vi "AprilTag Target Package Code 1.vi"() -> ()   [LabVIEW 2023]
uses:
  Camera Info.ctl
  State Machine/AprialTag Main Cluster.ctl
  State Machine/AprialTag States.ctl
  <vilib>/vision/Image Controls.llb/IMAQ Image.ctl
  Steam Type.ctl
  Camera Set Up/Event Setup Types.ctl
  <vilib>/Utility/config.llb/Read Key (String).vi
  <vilib>/Utility/config.llb/Write Key (String).vi
  <vilib>/Utility/config.llb/NI_LVConfig.lvlib
panel:
  in  "Main":enum32{"Page 1", "Page 2"}(tab)
  out "Target Pitch":dbl[](array[numeric]) caption="Tag Pitch (deg)" format="%.1f"
  out "Target Yaw":dbl[](array[numeric]) caption="Tag Yaw (deg)" format="%.1f"
  out "Tag ID":dbl[](array[numeric]) caption="Tag Number"
  out "Image":T1(plugin-control)
  in  "Camera Name":string="cam0"
  in  "Settings":bool
  in  "Save":bool
  in  "Tools":bool
  out "AprilTag Fps":dbl format="%#.0f"
  out "Distance":dbl[](array[numeric]) caption="Tag Distance (in)" format="%.1f"
  out "Angle":dbl[](array[numeric]) caption="Center Angle (deg)" format="%.1f"
  in  "Home":bool
  in  "Robot Calibration Cluster":T2={"Camera Height on robot (in)"=9.5, "Camera Angle on the robot (deg)"=2.5, "Camera FOV Top to Bottom View Angle (deg)"=26.5, "Camera FOV Left to Right View Angle (deg)"=68.5, "Target size (in)"=6.5, "Distance to front of bumper (in)"=9.75, "Focal Length (mm)"=10.0} {"Camera FOV Left to Right View Angle (deg)" format="%#_13g"; "Focal Length (mm)" format="%#_13g"; "Distance to front of bumper (in)" format="%#_13g"; "Target size (in)" format="%#_13g"; "Camera FOV Top to Bottom View Angle (deg)" format="%#_13g"; "Camera Angle on the robot (deg)" format="%#_13g"; "Camera Height on robot (in)" format="%#_13g"}
  # "Edit the camera name to the camera that you are going to use for this target package"
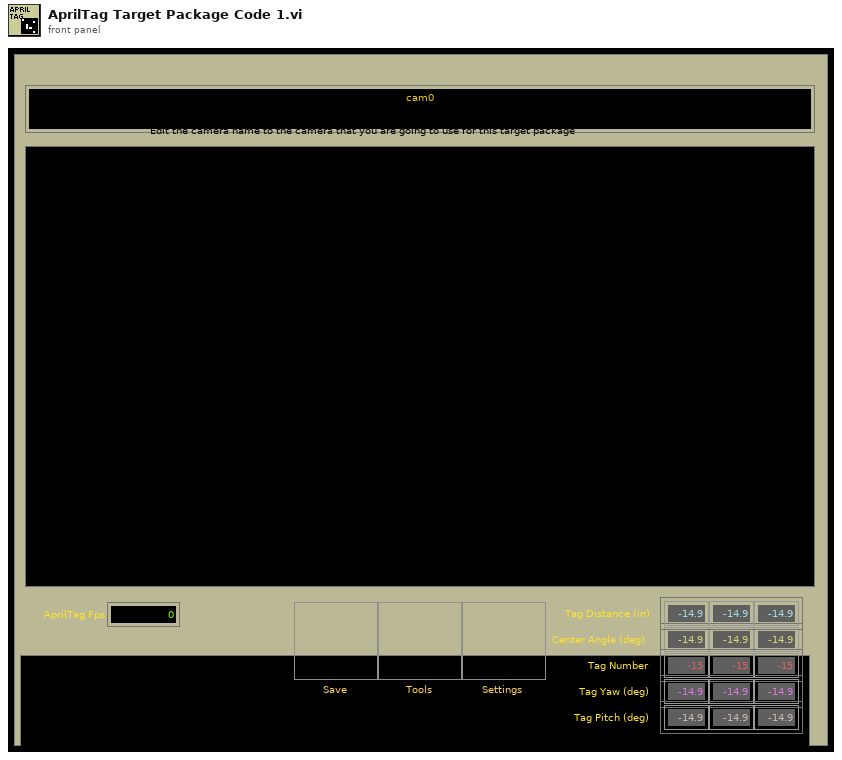
[diagram p1: front panel]
types:
  T1 = typedef "IMAQ Image.ctl" = refnum<image>
  T2 = typedef "Camera Info.ctl" = cluster{"Camera Height on robot (in)":dbl, "Camera Angle on the robot (deg)":dbl, "Camera FOV Top to Bottom View Angle (deg)":dbl, "Camera FOV Left to Right View Angle (deg)":dbl, "Target size (in)":dbl, "Distance to front of bumper (in)":dbl, "Focal Length (mm)":dbl}
  T3 = typedef "AprialTag States.ctl" = enum16{"Message Dispatcher", "INI", "Open", "Save", "Exit"}
  T4 = typedef "AprialTag Main Cluster.ctl" = cluster{"AprilTage FIFO":T3[], "Camera Name":string, "AprilTag path":path, "Control Ref's":refnum<vi>[], "Calibration Mask":T1, "Main Image":T1, "Timeout":i32, "EDIT Settings":bool, "Calibration path":path, "Camera Number":dbl}
  T5 = typedef "Steam Type.ctl" = enum8{"Unknown", "Apriltag", "Algae", "Coral"}
  T6 = typedef "Event Setup Types.ctl" = enum16{"Default", "Camera Loop Started", "Close Settings", "GreyScale", "Open Front Panel", "Save Data", "Exit"}
  T7 = cluster{"tag ID":i32, "Center":cluster{"X":dbl, "Y":dbl}, "homography matrix":dbl[], "decision margin":dbl, "Hamming Dist":i32, "corner points":cluster{"X":dbl, "Y":dbl}[], "Tag Family":string}[]
  T8 = typedef "AprilTag Target Fields.ctl" = cluster{"diameter points":cluster{"first point":cluster{"x":dbl, "y":dbl}, "projected point":cluster{"x":dbl, "y":dbl}}, "normalized center":cluster{"x":dbl, "y":dbl}, "Overall Score":dbl, "Distance (ft)":dbl, "Offset Angle":dbl, "Tag corner points":cluster{"X":dbl, "Y":dbl}[], "Tag Center":cluster{"X":dbl, "Y":dbl}, "Tag Yaw":dbl, "Tag Pitch":dbl, "Target Roll (deg)":dbl, "AprilTag Number":i32}
  T9 = typedef "Image Type" = u32
  T10 = typedef "NI_LVConfig.lvlib/Config Data RefNum.ctl" = refnum<k1>
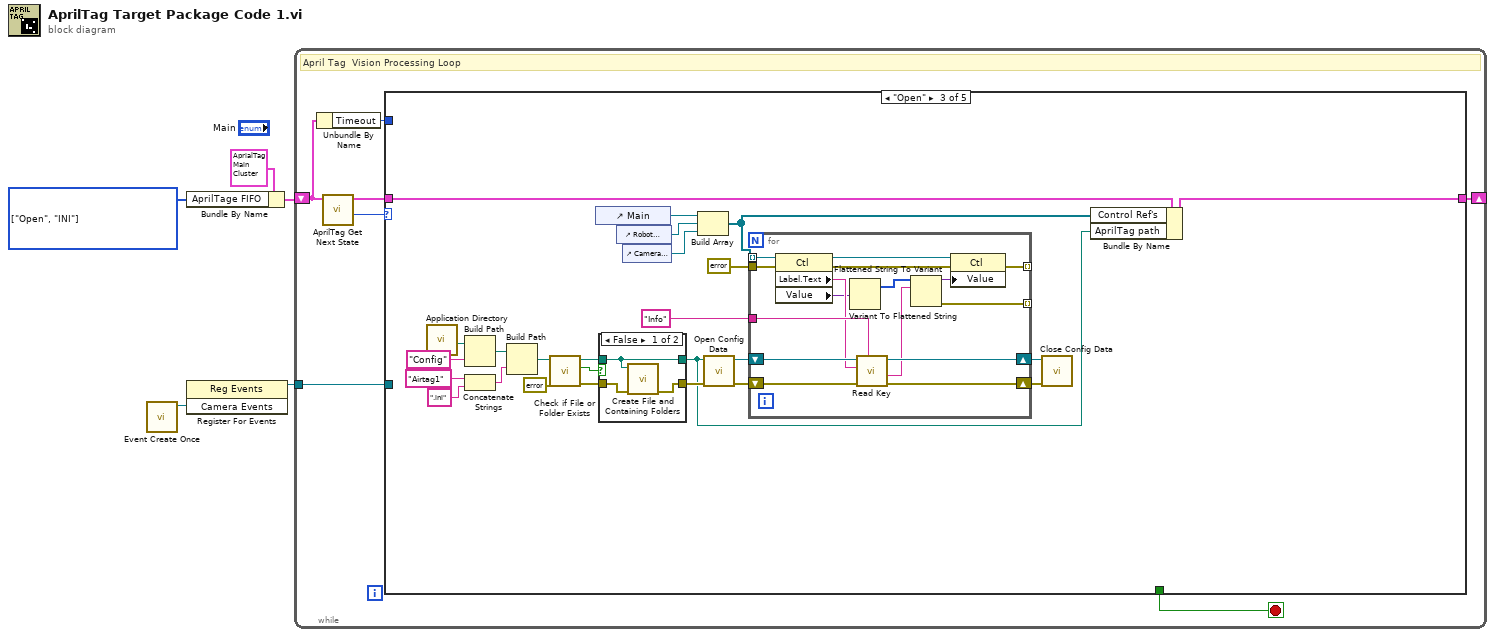
[diagram p0: block diagram]
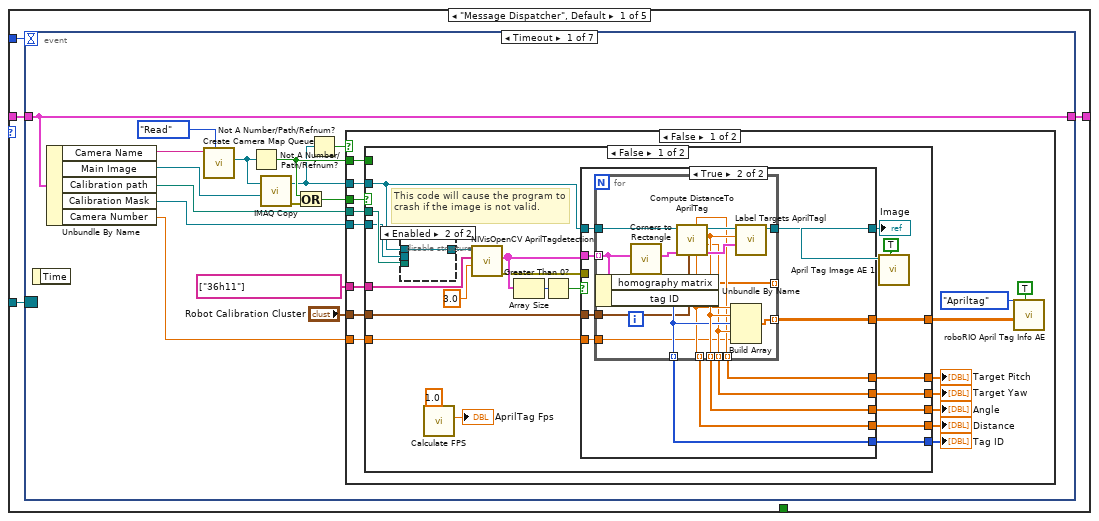
[diagram p2: hidden frame]
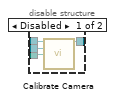
[diagram p3: hidden frame]
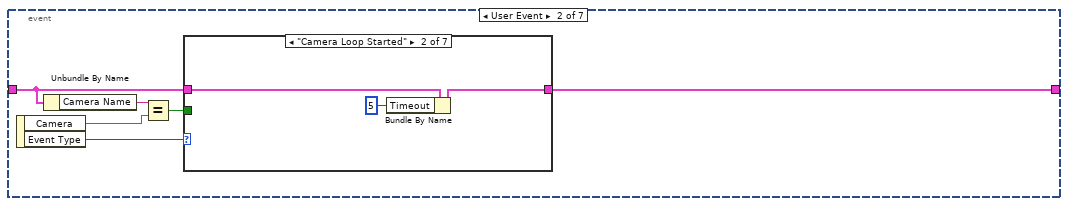
[diagram p7: hidden frame]
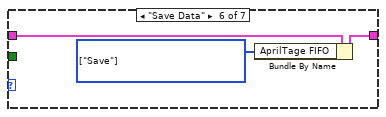
[diagram p12: hidden frame]
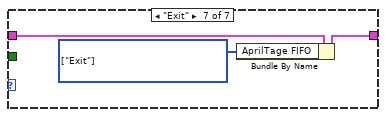
[diagram p13: hidden frame]
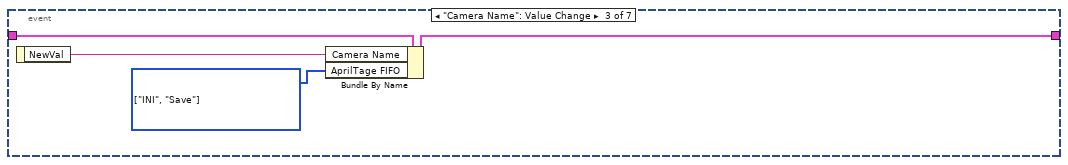
[diagram p14: hidden frame]
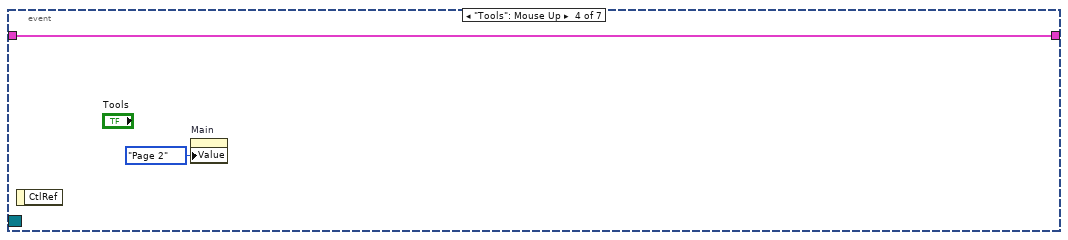
[diagram p15: hidden frame]
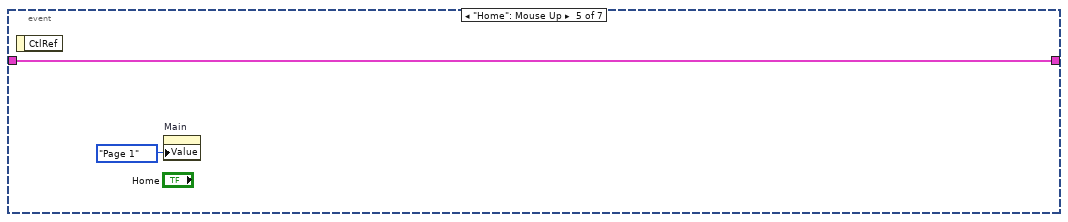
[diagram p16: hidden frame]
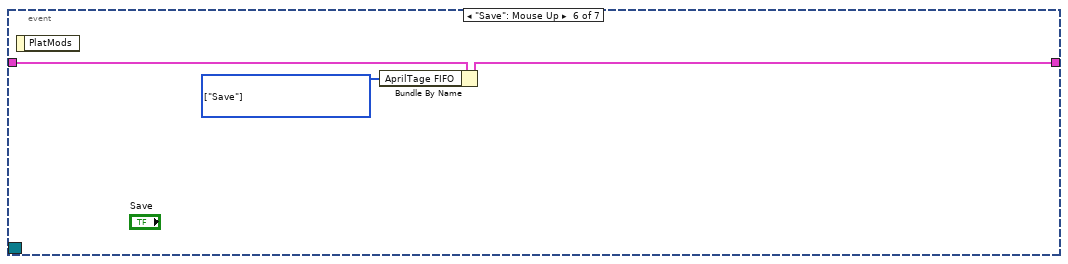
[diagram p17: hidden frame]
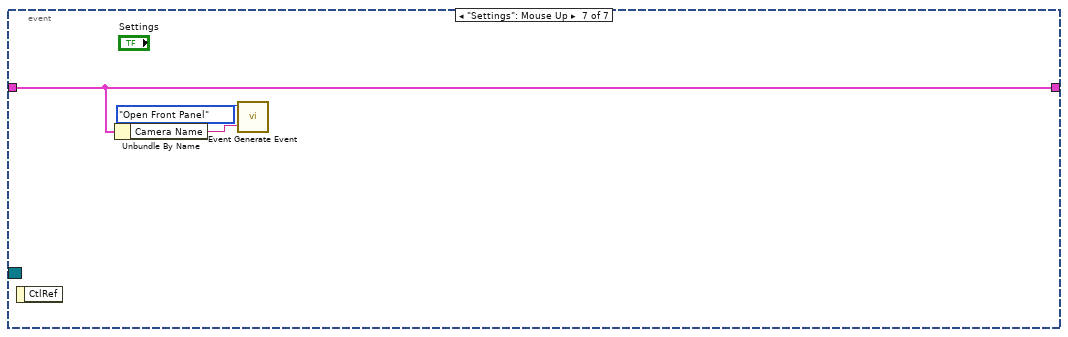
[diagram p18: hidden frame]
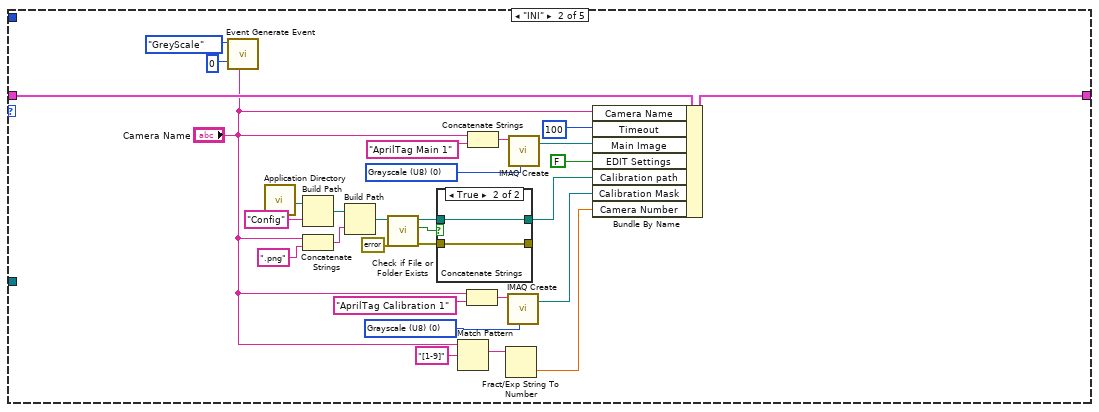
[diagram p19: hidden frame]
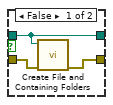
[diagram p20: hidden frame]
diagram:
  w1 = T3[] [enum."Open", enum."INI"] items=["Message Dispatcher", "INI", "Open", "Save", "Exit"] ("AprilTage FIFO")
  n1 = call "Event Create Once.vi"() -> ("Camera Events"=w5:refnum<user-event>)  [unwired: 10 in, 1 out]
  n2 = Bundle By Name(cluster=T4 {"AprilTage FIFO"=[], "Camera Name"="", "AprilTag path"=path "", "Control Ref's"=[], "Calibration Mask"=refnum, "Main Image"=refnum, "Timeout"=5, "EDIT Settings"=FALSE, "Calibration path"=path "", "Camera Number"=0.0} ("AprilTag Main Cluster out"), "AprilTage FIFO"=w1) -> (w2:T4)
  n3 = register-events(w5) -> (reference out=w4:refnum<event-registration>)  [unwired: 2 in, 1 out]
  n4 = while {
    tunnel: w4 -> [w12]
    shift-right: [w8] -> _
    shift-left: w2 -> [w6]
    stop <- w11 stop-if-true
    # "April Tag  Vision Processing Loop"
    n5 = Unbundle By Name(w6) -> ("Timeout"=w7:i32)
    n6 = call "AprilTag Get Next State.vi"("AprilTag Main Cluster in"=w6) -> ("Next State"=w9:T3, "AprilTag Main Cluster out"=w10:T4)  [unwired: 9 in]
    n7 = case shown="\"Open\"" w9 {
      tunnel: w12 -> [w16 _ _ _ _]
      tunnel: [_ _ _ _ TRUE] -> w11
      tunnel: w10 -> [w14 w163 w180 w218 w235]
      tunnel: [w15 w162 w178 w218 w235] -> w8
      tunnel: w7 -> [w13 _ _ _ _]
      frame "Message Dispatcher", Default {
        n8 = event shown="[0] Timeout" {
          selector: w16 -> [_ _ _ _ _ _ _]
          dyn-events: _ -> [_ _ _ _ _ _ _]
          timeout: w13 -> [_ _ _ _ _ _ _]
          tunnel: w14 -> [w31 w105 w124 w125 w127 w131 w133]
          tunnel: [w31 w107 w123 w125 w127 w130 w133] -> w15
          event Timeout {
            n9 = event-data() -> ()  [unwired: 1 in, 1 out]
            n10 = Unbundle By Name(w31) -> ("Camera Name"=w25:string, "Main Image"=w21:T1, "Calibration path"=w30:path, "Calibration Mask"=w18:T1, "Camera Number"=w17:dbl)
            n11 = call "Create Camera Map Queue.vi"("Action"=enum16{"Read", "Write"}."Read", "Camera"=w25) -> ("Image out"=w24:T1)  [unwired: 8 in, 1 out]
            n12 = Not A Number/Path/Refnum?(number/path/refnum=w24) -> (NaN/Path/Refnum?=w27:bool)
            n13 = call "IMAQ Copy"("Image Dst"=w21, "Image Src"=w24) -> ("error out"=w22:errorcluster, "Image Dst Out"=w19:T1)  [unwired: 4 in]
            n14 = Or(x=w27, y=w22) -> (x .or. y?=w23:bool)
            n15 = Not A Number/Path/Refnum?(number/path/refnum=w19) -> (NaN/Path/Refnum?=w20:bool)
            n16 = case shown="False" w20 {
              tunnel: w30 -> [w44 _]
              tunnel: string[] ["36h11"] ("Tag Familys") -> [w43 _]
              tunnel: "Robot Calibration Cluster" -> [w42 _]
              tunnel: w27 -> [w41 _]
              tunnel: w23 -> [w35 _]
              tunnel: w19 -> [w34 _]
              tunnel: w18 -> [w33 _]
              tunnel: w17 -> [w32 _]
              frame False {
                n17 = case shown="False" w35 {
                  tunnel: w43 -> [w69 _]
                  tunnel: w42 -> [w68 _]
                  tunnel: [w59 _] -> w46
                  tunnel: w41 -> [_ _]
                  tunnel: w44 -> [w52 _]
                  tunnel: [w58 _] -> w40
                  tunnel: [w57 _] -> w39
                  tunnel: [w56 _] -> w38
                  tunnel: [w55 _] -> w37
                  tunnel: [w54 _] -> w36
                  tunnel: w34 -> [w51 _]
                  tunnel: w33 -> [w49 _]
                  tunnel: w32 -> [w48 _]
                  frame False {
                    # "This code will cause the program to crash if the image is not valid."
                    n18 = disable-structure shown="Enabled" {
                      disable-tunnel: w52 -> [w73 _]
                      disable-tunnel: w51 -> [w72 w74]
                      disable-tunnel: [w71 w74] -> w50
                      disable-tunnel: w49 -> [w70 _]
                      frame Disabled {
                        n19 = call "Calibrate Camera.vi"("Image In"=w72, "Image Dst"=w70, "File Path (Image Calibration 1)"=w73) -> ("Image Out"=w71:T1)  [unwired: 10 in, 2 out]
                      }
                      frame Enabled {
                      }
                    }
                    n20 = call "Calculate FPS.vi"("Frames Processed"=1.0) -> ("Fps"=→"AprilTag Fps":dbl)  [unwired: 10 in]
                    n21 = call "NIVisOpenCV AprilTagdetection.vi"("decimate"=3.0, "Tag Familys"=w69, "Image Src"=w50) -> ("error out"=w64:errorcluster, "Detected Tags"=w67:T7)  [unwired: 5 in, 2 out]
                    n22 = Array Size(array=w67) -> (size(s)=w66:i32)
                    n23 = Greater Than 0?(x=w66) -> (x > 0?=w65:bool)
                    n24 = case shown="True" w65 {
                      tunnel: w51 -> [w75 w86]
                      tunnel: w67 -> [_ w85]
                      tunnel: [w75 w84] -> w63
                      tunnel: w64 -> [_ _]
                      tunnel: w68 -> [_ w83]
                      tunnel: [_ w82] -> w59
                      tunnel: [_ w81] -> w58
                      tunnel: [_ w80] -> w57
                      tunnel: [_ w79] -> w56
                      tunnel: [_ w78] -> w55
                      tunnel: [_ w77] -> w54
                      tunnel: w48 -> [_ w76]
                      frame False {
                      }
                      frame True {
                        n25 = for {
                          tunnel: w85 -> [w99] mode=indexing
                          tunnel: w86 -> [w100]
                          tunnel: [w101] -> w84
                          tunnel: [w94] -> w79 mode=indexing
                          tunnel: [w92] -> w77 mode=indexing
                          tunnel: [w95] -> w78 mode=indexing
                          tunnel: w83 -> [w93]
                          tunnel: [w91] -> w80 mode=indexing
                          tunnel: [w90] -> w82 mode=indexing
                          tunnel: [w89] -> w81 mode=indexing
                          tunnel: w76 -> [w88]
                          tunnel: [w87] -> _ mode=indexing
                          n26 = Unbundle By Name(w99) -> ("homography matrix"=w87:dbl[], "tag ID"=w94:i32)
                          n27 = call "Corners to Rectangle.vi"("tag info"=w99) -> ("output cluster"=w98:T8)  [unwired: 10 in]
                          n28 = call "Compute DistanceTo AprilTag.vi"("Robot Calibration Cluster"=w93, "results"=w98, "Image Src"=w100) -> ("results out"=w97:T8, "Target Yaw (deg)"=w91:dbl, "Offset Angle"=w95:dbl, "Image Dst Out"=w96:T1, "Distance from target (in)"=w92:dbl, "Target Pitch (deg)"=w89:dbl)  [unwired: 3 in]
                          n29 = Build Array(w92, w95, w94, w91, w88) -> (w90:dbl[])
                          n30 = call "Label Targets AprilTagl.vi"("results"=w97, "Angle"=w95, "Image in"=w96) -> ("Image out"=w101:T1)  [unwired: 8 in]
                        }
                      }
                    }
                    "Image" <- w63
                    n31 = call "April Tag Image AE 1.vi"("Update"=TRUE, "Ball Image in"=w63) -> ()  [unwired: 9 in, 1 out]
                  }
                  frame True {
                  }
                }
                "Distance" <- w36
                "Angle" <- w37
                "Tag ID" <- w38
                "Target Yaw" <- w39
                "Target Pitch" <- w40
                n32 = call "roboRIO April Tag Info AE.vi"("Update"=TRUE, "Info in"=w46, "Stream Type"=Steam_Type."Apriltag") -> ()  [unwired: 8 in, 1 out]
              }
              frame True {
              }
            }
          }
          event User Event {
            n33 = event-data() -> ("Camera"=w103:string, "Event Type"=w106:T6)  [unwired: 1 in]
            n34 = Unbundle By Name(w105) -> ("Camera Name"=w104:string)
            n35 = Equal?(x=w104, y=w103) -> (x = y?=w102:bool)
            n36 = case shown="\"Camera Loop Started\"" w106 {
              tunnel: w105 -> [w108 w111 w112 w113 w114 w117 w120]
              tunnel: [w108 w110 w112 w113 w114 w116 w119] -> w107
              tunnel: w102 -> [_ _ _ _ _ _ _]
              frame "Default" {
              }
              frame "Camera Loop Started" {
                n37 = Bundle By Name(cluster=w111, "Timeout"=5) -> (w110:T4)
              }
              frame "Close Settings" {
              }
              frame "GreyScale" {
              }
              frame "Open Front Panel" {
              }
              frame "Save Data" {
                w115 = T3[] [enum."Save"] items=["Message Dispatcher", "INI", "Open", "Save", "Exit"] ("AprilTage FIFO")
                n38 = Bundle By Name(cluster=w117, "AprilTage FIFO"=w115) -> (w116:T4)
              }
              frame "Exit" {
                w118 = T3[] [enum."Exit"] items=["Message Dispatcher", "INI", "Open", "Save", "Exit"] ("AprilTage FIFO")
                n39 = Bundle By Name(cluster=w120, "AprilTage FIFO"=w118) -> (w119:T4)
              }
            }
          }
          event "Camera Name": Value Change {
            w122 = T3[] [enum."INI", enum."Save"] items=["Message Dispatcher", "INI", "Open", "Save", "Exit"] ("AprilTage FIFO")
            n40 = event-data() -> ("NewVal"=w121:string)  [unwired: 1 in]
            n41 = Bundle By Name(cluster=w124, "Camera Name"=w121, "AprilTage FIFO"=w122) -> (w123:T4)
          }
          event "Tools": Mouse Up {
            n42 = event-data() -> ()  [unwired: 1 in, 1 out]
            n43 = property on="Main" class="TabCtl (strict)"("Value"=enum32{"Page 1", "Page 2"}."Page 2" ("Main")) -> ()  [unwired: 2 in, 2 out]
          }
          event "Home": Mouse Up {
            n44 = event-data() -> ()  [unwired: 1 in, 1 out]
            n45 = property on="Main" class="TabCtl (strict)"("Value"=enum32{"Page 1", "Page 2"}."Page 1" ("Main")) -> ()  [unwired: 2 in, 2 out]
          }
          event "Save": Mouse Up {
            w129 = T3[] [enum."Save"] items=["Message Dispatcher", "INI", "Open", "Save", "Exit"] ("AprilTage FIFO")
            n46 = event-data() -> ()  [unwired: 1 in, 1 out]
            n47 = Bundle By Name(cluster=w131, "AprilTage FIFO"=w129) -> (w130:T4)
          }
          event "Settings": Mouse Up {
            n48 = event-data() -> ()  [unwired: 1 in, 1 out]
            n49 = Unbundle By Name(w133) -> ("Camera Name"=w132:string)
            n50 = call "Event Generate Event.vi"("Camera Name"=w132, "Event Type"=Event_Setup_Types."Open Front Panel") -> ()  [unwired: 10 in]
          }
        }
      }
      frame "INI" {
        w139 = T9 0 items=["Grayscale (U8)", "Grayscale (I16)", "Grayscale (SGL)", "Complex (CSG)", "RGB (U32)", "HSL (U32)", "RGB (U64)", "Grayscale (U16)"] ("Image Type")
        w160 = T9 0 items=["Grayscale (U8)", "Grayscale (I16)", "Grayscale (SGL)", "Complex (CSG)", "RGB (U32)", "HSL (U32)", "RGB (U64)", "Grayscale (U16)"] ("Image Type")
        n51 = call "Event Generate Event.vi"("Camera Name"="Camera Name", "Setpoint"=i64 0, "Event Type"=Event_Setup_Types."GreyScale") -> ()  [unwired: 9 in]
        n52 = call <vilib>:"Application Directory.vi"() -> ("Application Directory"=w153:path)
        n53 = Build Path(base path=w153, name or relative path="Config") -> (appended path=w151:path)
        n54 = Concatenate Strings("Camera Name", ".png" ("name or relative path")) -> (w155:string)
        n55 = Build Path(base path=w151, name or relative path=w155) -> (appended path=w150:path)
        n56 = call <vilib>:"Check if File or Folder Exists.vi"("error in (no error)"=errorcluster {"status"=FALSE, "code"=0, "source"=""}, "path"=w150) -> ("error out"=w147:errorcluster, "file or folder exists?"=w148:bool, "dup path"=w149:path)  [unwired: 7 in]
        n57 = case shown="True" w148 {
          tunnel: [w166 w167] -> _
          tunnel: w149 -> [w165 w168]
          tunnel: [w165 w168] -> w145
          tunnel: w147 -> [w164 w167]
          frame False {
            n58 = call <vilib>:"Create File and Containing Folders.vi"("error in (no error)"=w164, "file path"=w165) -> ("error out"=w166:errorcluster)  [unwired: 8 in, 1 out]
          }
          frame True {
          }
        }
        n59 = Match Pattern(string="Camera Name", regular expression="[1-9]") -> (match substring=w136:string)  [unwired: 1 in, 3 out]
        n60 = Concatenate Strings("Camera Name", "AprilTag Calibration 1" ("string")) -> (w141:string)
        n61 = Concatenate Strings("Camera Name", "AprilTag Main 1" ("string")) -> (w159:string)
        n62 = Fract/Exp String To Number(string=w136) -> (number=w135:dbl)  [unwired: 3 in, 1 out]
        n63 = call "IMAQ Create"("Image Name"=w141, "Image Type"=w139) -> ("New Image"=w140:T1)  [unwired: 2 in, 2 out]
        n64 = call "IMAQ Create"("Image Name"=w159, "Image Type"=w160) -> ("New Image"=w157:T1)  [unwired: 2 in, 2 out]
        n65 = Bundle By Name(cluster=w163, "Camera Name"="Camera Name", "Timeout"=100, "Main Image"=w157, "EDIT Settings"=FALSE, "Calibration path"=w145, "Calibration Mask"=w140, "Camera Number"=w135) -> (w162:T4)
      }
      frame "Open" {
        n66 = call <vilib>:"Application Directory.vi"() -> ("Application Directory"=w183:path)
        n67 = Build Path(base path=w183, name or relative path="Config") -> (appended path=w181:path)
        n68 = Concatenate Strings("Airtag1" ("string"), ".ini" ("name or relative path")) -> (w193:string)
        n69 = Build Path(base path=w181, name or relative path=w193) -> (appended path=w174:path)
        n70 = call <vilib>:"Check if File or Folder Exists.vi"("error in (no error)"=errorcluster {"status"=FALSE, "code"=0, "source"=""}, "path"=w174) -> ("error out"=w170:errorcluster, "file or folder exists?"=w172:bool, "dup path"=w173:path)  [unwired: 7 in]
        n71 = control-ref of="Main"() -> (w188:refnum<vi>)
        n72 = case shown="False" w172 {
          tunnel: [w196 w197] -> w184
          tunnel: w173 -> [w195 w198]
          tunnel: [w195 w198] -> w171
          tunnel: w170 -> [w194 w197]
          frame False {
            n73 = call <vilib>:"Create File and Containing Folders.vi"("error in (no error)"=w194, "file path"=w195) -> ("error out"=w196:errorcluster)  [unwired: 8 in, 1 out]
          }
          frame True {
          }
        }
        n74 = control-ref of="Robot Calibration Cluster"() -> (w187:refnum<vi>)
        n75 = control-ref of="Camera Name"() -> (w179:refnum<vi>)
        n76 = Build Array(w188, w187, w179) -> (w177:refnum<vi>[])
        n77 = call <vilib>:"Open Config Data.vi"("error in (no error)"=w184, "configuration file path"=w171) -> ("error out"=w189:errorcluster, "refnum"=w192:T10)  [unwired: 7 in, 1 out]
        n78 = for {
          tunnel: "Info" ("Camera Name") -> [w211]
          tunnel: w177 -> [w209] mode=indexing
          shift-right: [w213] -> w191
          shift-left: w192 -> [w214]
          shift-right: [w212] -> w190
          shift-left: w189 -> [w210]
          tunnel: [w204] -> _ mode=indexing
          tunnel: errorcluster {"status"=FALSE, "code"=0, "source"=""} ("error out") -> [w203]
          tunnel: [w199] -> _ mode=indexing
          n79 = property class="Ctl"(reference=w209, error in=w203) -> (reference out=w207:refnum<vi>, error out=w205:errorcluster, "Label.Text"=w208:string, "Value"=w201:variant)
          n80 = Variant To Flattened String(Variant=w201) -> (1:w200:i16[])  [unwired: 1 out]
          n81 = call-poly <vilib>:"Read Key.vi"("section"=w211, "error in (no error)"=w210, "key"=w208, "refnum"=w214) -> ("error out"=w212:errorcluster, "value"=w206:string, "refnum out"=w213:T10)  [unwired: 4 in, 1 out]
          n82 = Flattened String To Variant(6:w206, 7:w200) -> (0:w199:errorcluster, 3:w202:variant)  [unwired: 1 in]
          n83 = property class="Ctl"(reference=w207, error in=w205, "Value"=w202) -> (error out=w204:errorcluster)  [unwired: 1 out]
        }
        n84 = call <vilib>:"Close Config Data.vi"("error in (no error)"=w190, "refnum"=w191) -> ()  [unwired: 8 in, 2 out]
        n85 = Bundle By Name(cluster=w180, "Control Ref's"=w177, "AprilTag path"=w171) -> (w178:T4)
      }
      frame "Save" {
        n86 = Unbundle By Name(w218) -> ("Control Ref's"=w216:refnum<vi>[], "AprilTag path"=w217:path)
        n87 = call <vilib>:"Open Config Data.vi"("configuration file path"=w217) -> ("error out"=w219:errorcluster, "refnum"=w222:T10)  [unwired: 8 in, 1 out]
        n88 = for {
          tunnel: "Info" ("Camera Name") -> [w228]
          shift-right: [w231] -> w221
          shift-left: w222 -> [w232]
          shift-right: [w230] -> w220
          shift-left: w219 -> [w229]
          tunnel: w216 -> [w223] mode=indexing
          n89 = property class="Ctl"(reference=w223, error in=w229) -> (error out=w225:errorcluster, "Label.Text"=w227:string, "Value"=w226:variant)  [unwired: 1 out]
          n90 = Variant To Flattened String(Variant=w226) -> (data string=w224:string)  [unwired: 1 out]
          n91 = call-poly <vilib>:"Write Key.vi"("section"=w228, "error in (no error)"=w225, "value"=w224, "key"=w227, "refnum"=w232) -> ("error out"=w230:errorcluster, "refnum out"=w231:T10)  [unwired: 4 in, 1 out]
        }
        n92 = call <vilib>:"Close Config Data.vi"("error in (no error)"=w220, "refnum"=w221) -> ()  [unwired: 8 in, 2 out]
      }
      frame "Exit" {
        n93 = Unbundle By Name(w235) -> ("Calibration Mask"=w234:T1, "Main Image"=w233:T1)
        n94 = call "IMAQ Dispose"("Image"=w234) -> ()  [unwired: 5 in, 1 out]
        n95 = call "IMAQ Dispose"("Image"=w233) -> ()  [unwired: 5 in, 1 out]
      }
    }
  }
